vi "Get VIs in Project.vi"(8 "error in (no error)":errorcluster, 11 "project":refnum<vi>) -> (0 "error out":errorcluster, 2 "Array of VIs":T2(array[cluster]), 3 "project out":refnum<vi>)   [LabVIEW 2017, in "csm-file-support.lvlib"]
uses:
  csm-file-support.lvlib
  <vilib>/addons/analyzer/_analyzerctrls.llb/VIAnCtl Analysis App Info.ctl
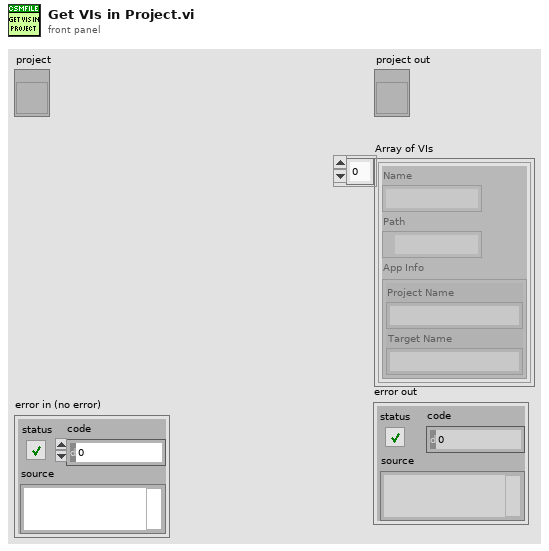
[diagram p1: front panel]
types:
  T1 = typedef "VIAnCtl Analysis App Info.ctl" = cluster{"Project Name":string, "Target Name":string}
  T2 = cluster{"Name":string, "Path":path, "App Info":T1}[]
  T3 = cluster{"Name":string, "Path":path, "App Info":T1}
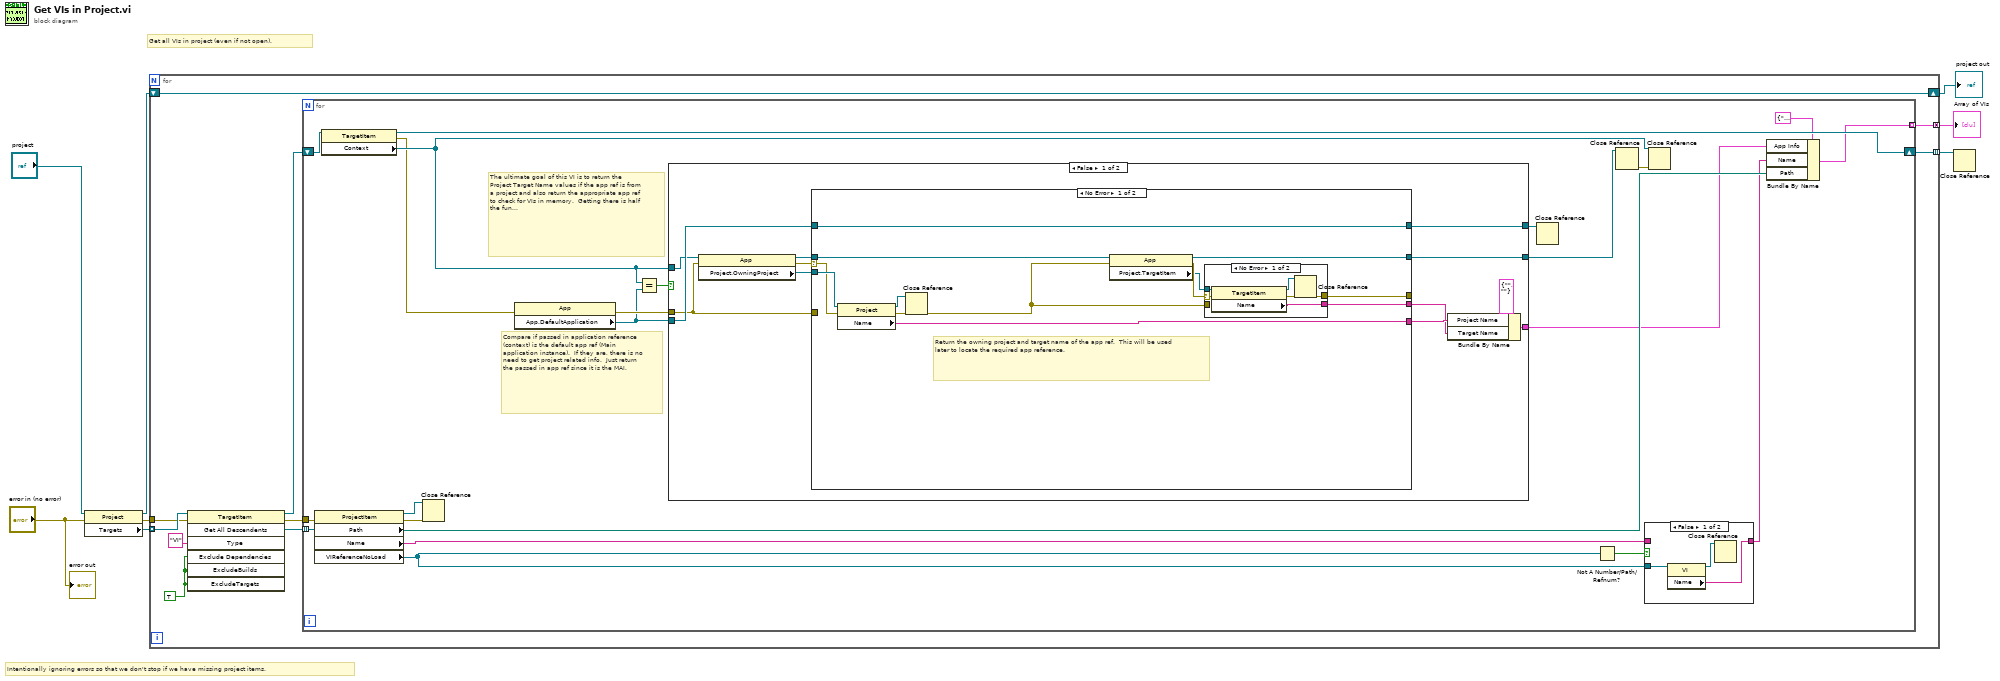
[diagram p0: block diagram]
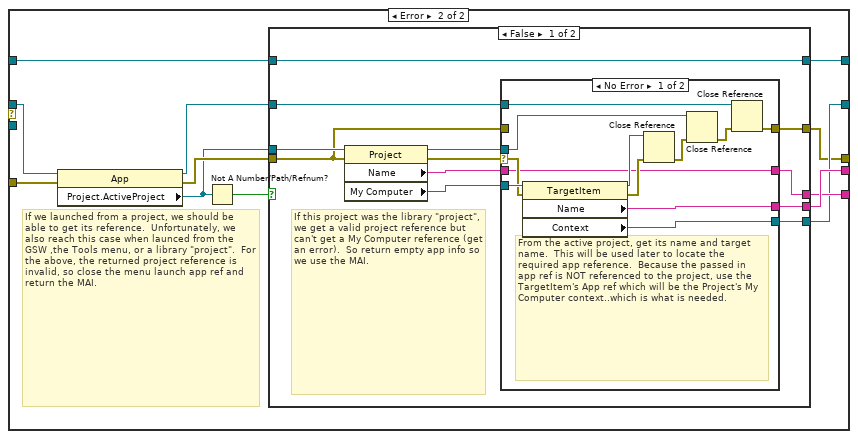
[diagram p3: hidden frame]
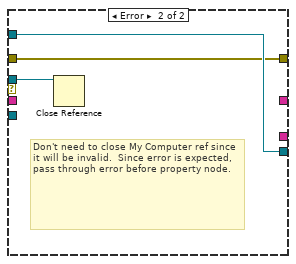
[diagram p4: hidden frame]
diagram:
  # "Intentionally ignoring errors so that we don't stop if we have missing project items."
  # "Get all VIs in project (even if not open)."
  n1 = property class="Project"(reference="project", error in="error in (no error)") -> (reference out=w2:refnum<vi>, error out=w6:errorcluster, "Targets"=w8:refnum<vi>[])
  n2 = for {
    tunnel: w8 -> [w18] mode=indexing
    tunnel: [w12] -> w5 mode=indexing
    tunnel: [w11] -> w4 mode=concatenating
    tunnel: w6 -> [w15]
    shift-right: [w9] -> w1
    shift-left: w2 -> [w9]
    w10 = TRUE ("ExcludeDependencies")
    n3 = invoke class="TargetItem" method="Get All Descendents"(reference=w18, error in=w15, "Type"="VI", "Exclude Dependencies"=w10, "ExcludeBuilds"=w10, "ExcludeTargets"=w10) -> (reference out=w13:refnum<vi>, error out=w14:errorcluster, "All Descendents"=w16:refnum<vi>[])  [unwired: 1 in, 4 out]
    n4 = for {
      tunnel: w16 -> [w40] mode=indexing
      shift-right: [w35] -> w12
      shift-left: w13 -> [w36]
      tunnel: [w32] -> w11 mode=indexing
      tunnel: w14 -> [w39]
      # "Compare if passed in application reference (context) is the default app ref (Main application instance).  If they are, there is no need to get project related info.  Just return the passed in app ref since it is the MAI."
      # "The ultimate goal of this VI is to return the Project Target Name values if the app ref is from a project and also return the appropriate app ref to check for VIs in memory.  Getting there is half the fun..."
      n5 = property class="ProjectItem"(reference=w40, error in=w39) -> (reference out=w37:refnum<vi>, error out=w38:errorcluster, "Path"=w33:path, "Name"=w30:string, "VIReferenceNoLoad"=w29:refnum<vi>)
      n6 = property class="TargetItem"(reference=w36) -> (reference out=w35:refnum<vi>, error out=w19:errorcluster, "Context"=w24:refnum<vi>)  [unwired: 1 in]
      n7 = Close Reference(reference=w37, error in (no error)=w38) -> ()  [unwired: 1 out]
      n8 = property class="App"(error in=w19) -> (error out=w23:errorcluster, "App.DefaultApplication"=w22:refnum<vi>)  [unwired: 1 in, 1 out]
      n9 = Equal?(x=w24, y=w22) -> (x = y?=w21:bool)
      n10 = case shown="False" w21 {
        tunnel: w23 -> [w41 _]
        tunnel: [w52 w116] -> w26
        tunnel: [w51 _] -> w27
        tunnel: w24 -> [w45 w116]
        tunnel: w22 -> [w47 w115]
        tunnel: [w46 w115] -> w20
        frame False {
          n11 = property class="App"(reference=w45, error in=w41) -> (reference out=w43:refnum<vi>, error out=w42:errorcluster, "Project.OwningProject"=w44:refnum<vi>)
          n12 = case shown="No Error" w42 {
            selector: w42 -> [w54 _]
            tunnel: [w65 w77] -> _
            tunnel: [w64 w78] -> w52
            tunnel: [w58 w80] -> w49
            tunnel: [w57 w81] -> w48
            tunnel: w44 -> [w56 _]
            tunnel: w43 -> [w55 w83]
            tunnel: w41 -> [_ w84]
            tunnel: w47 -> [w53 w74]
            tunnel: [w53 w73] -> w46
            frame No Error {
              # "Return the owning project and target name of the app ref.  This will be used later to locate the required app reference."
              n13 = property class="Project"(reference=w56, error in=w54) -> (reference out=w62:refnum<vi>, error out=w63:errorcluster, "Name"=w58:string)
              n14 = Close Reference(reference=w62, error in (no error)=w63) -> (error out=w59:errorcluster)
              n15 = property class="App"(reference=w55, error in=w59) -> (reference out=w64:refnum<vi>, error out=w61:errorcluster, "Project.TargetItem"=w60:refnum<vi>)
              n16 = case shown="No Error" w61 {
                selector: w61 -> [w68 _]
                tunnel: w60 -> [w71 _]
                tunnel: [w67 w72] -> w65
                tunnel: [w66 _] -> w57
                tunnel: w59 -> [_ w72]
                frame No Error {
                  n17 = property class="TargetItem"(reference=w71, error in=w68) -> (reference out=w69:refnum<vi>, error out=w70:errorcluster, "Name"=w66:string)
                  n18 = Close Reference(reference=w69, error in (no error)=w70) -> (error out=w67:errorcluster)
                }
                frame Error {
                }
              }
            }
            frame Error {
              # "If we launched from a project, we should be able to get its reference.  Unfortunately, we also reach this case when launced from the GSW ,the Tools menu, or a library \"project\".  For the above, the returned project reference is invalid, so close the menu launch app ref and return the MAI."
              n19 = property class="App"(reference=w83, error in=w84) -> (reference out=w79:refnum<vi>, error out=w82:errorcluster, "Project.ActiveProject"=w76:refnum<vi>)
              n20 = Not A Number/Path/Refnum?(number/path/refnum=w76) -> (NaN/Path/Refnum?=w75:bool)
              n21 = case shown="False" w75 {
                tunnel: w82 -> [w85 w114]
                tunnel: [w94 _] -> w81
                tunnel: [w87 _] -> w80
                tunnel: w79 -> [w93 w112]
                tunnel: [w92 w113] -> w78
                tunnel: [w91 w114] -> w77
                tunnel: w76 -> [w90 _]
                tunnel: w74 -> [w86 w113]
                tunnel: [w86 w112] -> w73
                frame False {
                  # "If this project was the library \"project\", we get a valid project reference but can't get a My Computer reference (get an error).  So return empty app info so we use the MAI."
                  n22 = property class="Project"(reference=w90, error in=w85) -> (reference out=w96:refnum<vi>, error out=w89:errorcluster, "Name"=w88:string, "My Computer"=w95:refnum<vi>)
                  n23 = case shown="No Error" w89 {
                    selector: w89 -> [w98 _]
                    tunnel: w96 -> [w108 w111]
                    tunnel: w95 -> [w107 _]
                    tunnel: [w103 _] -> w94
                    tunnel: w93 -> [w102 w110]
                    tunnel: [w101 w110] -> w92
                    tunnel: [w99 w109] -> w91
                    tunnel: w88 -> [w97 _]
                    tunnel: [w97 _] -> w87
                    tunnel: w85 -> [_ w109]
                    frame No Error {
                      # "From the active project, get its name and target name.  This will be used later to locate the required app reference.  Because the passed in app ref is NOT referenced to the project, use the TargetItem's App ref which will be the Project's My Computer context..which is what is needed."
                      n24 = property class="TargetItem"(reference=w107, error in=w98) -> (reference out=w106:refnum<vi>, error out=w105:errorcluster, "Name"=w103:string, "Context"=w101:refnum<vi>)
                      n25 = Close Reference(reference=w106, error in (no error)=w105) -> (error out=w104:errorcluster)
                      n26 = Close Reference(reference=w108, error in (no error)=w104) -> (error out=w100:errorcluster)
                      n27 = Close Reference(reference=w102, error in (no error)=w100) -> (error out=w99:errorcluster)
                    }
                    frame Error {
                      # "Don't need to close My Computer ref since it will be invalid.  Since error is expected, pass through error before property node."
                      n28 = Close Reference(reference=w111) -> ()  [unwired: 1 in, 1 out]
                    }
                  }
                }
                frame True {
                }
              }
            }
          }
          n29 = Bundle By Name(cluster=T1 {"Project Name"="", "Target Name"=""} ("App Info"), "Project Name"=w49, "Target Name"=w48) -> (w51:T1)
        }
        frame True {
          # "For the MAI, app info is not applicable."
        }
      }
      n30 = Close Reference(reference=w20) -> ()  [unwired: 1 in, 1 out]
      n31 = Not A Number/Path/Refnum?(number/path/refnum=w29) -> (NaN/Path/Refnum?=w31:bool)
      n32 = Close Reference(reference=w26) -> (error out=w25:errorcluster)  [unwired: 1 in]
      n33 = case shown="False" w31 {
        tunnel: w30 -> [_ w120]
        tunnel: [w118 w120] -> w28
        tunnel: w29 -> [w119 _]
        frame False {
          n34 = property class="VI"(reference=w119) -> (reference out=w117:refnum<vi>, "Name"=w118:string)  [unwired: 1 in, 1 out]
          n35 = Close Reference(reference=w117) -> ()  [unwired: 1 in, 1 out]
        }
        frame True {
        }
      }
      n36 = Close Reference(reference=w24, error in (no error)=w25) -> ()  [unwired: 1 out]
      n37 = Bundle By Name(cluster=T3 {"Name"="", "Path"=path "", "App Info"={"Project Name"="", "Target Name"=""}}, "App Info"=w27, "Name"=w28, "Path"=w33) -> (w32:T3)
    }
  }
  "Array of VIs" <- w4
  "project out" <- w1
  n38 = Close Reference(reference=w5) -> ()  [unwired: 1 in, 1 out]
  "error out" <- "error in (no error)"
